vi "Start.vi"(8 "error in (no error)":errorcluster, 11 "Service Details":T1) -> (0 "error out":errorcluster, 3 "MicronTemplateAPIs out":refnum<class "MicronTemplateAPIs.lvclass">)   [LabVIEW 2019, in "MicronTemplateAPIs.lvlib" / "MicronTemplateAPIs.lvclass"]
uses:
  MicronTemplateAPIs.lvclass
  vi.lib/Micron/Base/Client/Typedefs/ServiceDetails.ctl
  vi.lib/Micron/Base/Client/MicronClient.lvclass
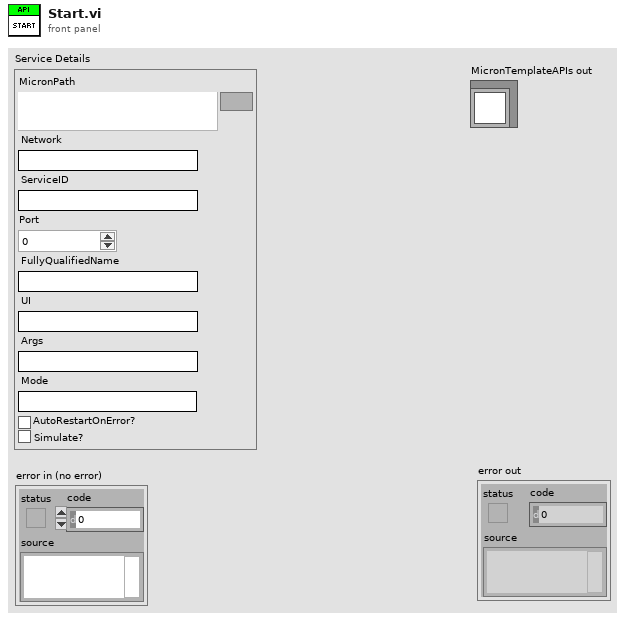
[diagram p1: front panel]
types:
  T1 = typedef "MicronClient.lvclass/ServiceDetails.ctl" = cluster{"MicronPath":path, "Network":string, "ServiceID":string, "Port":i32, "FullyQualifiedName":string, "UI":string, "Args":string, "Mode":string, "AutoRestartOnError?":bool, "Simulate?":bool}
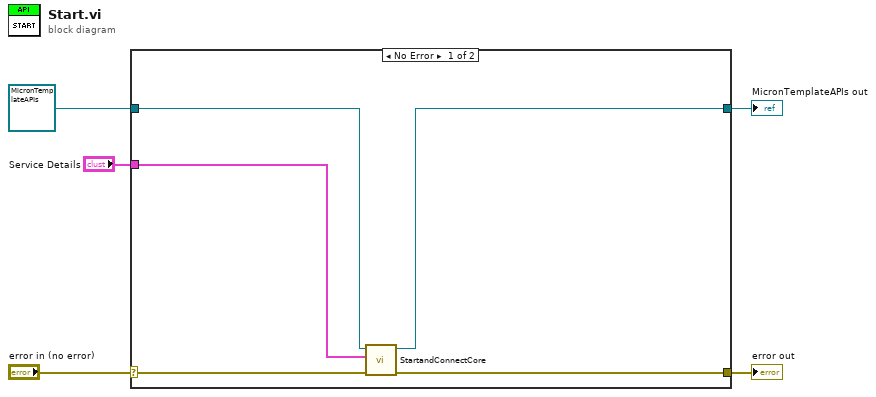
[diagram p0: block diagram]
diagram:
  n1 = case shown="No Error" "error in (no error)" {
    selector: "error in (no error)" -> [w10 w12]
    tunnel: [w9 w12] -> w4
    tunnel: [w7 w11] -> w2
    tunnel: refnum<class "MicronTemplateAPIs.lvclass"> refnum ("MicronTemplateAPIs in") -> [w8 w11]
    tunnel: "Service Details" -> [w6 _]
    frame No Error {
      n2 = call-dynamic "StartandConnectCore.vi"("error in (no error)"=w10, "Service Details"=w6, "MicronGRPCClient in"=w8) -> ("error out"=w9:errorcluster, "MicronGRPCClient out"=w7:refnum<class "MicronTemplateAPIs.lvclass">)  [unwired: 7 in]
    }
    frame Error {
    }
  }
  "error out" <- w4
  "MicronTemplateAPIs out" <- w2
